vi "GOOP_ExecuteDependencyViewerCommand.vi"(10 "Object":u64, 11 "Sub Command":string) -> ()   [LabVIEW 2020]
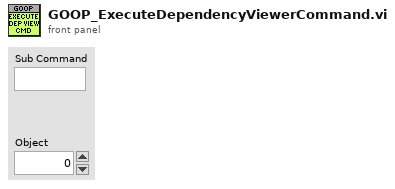
[diagram p1: front panel]
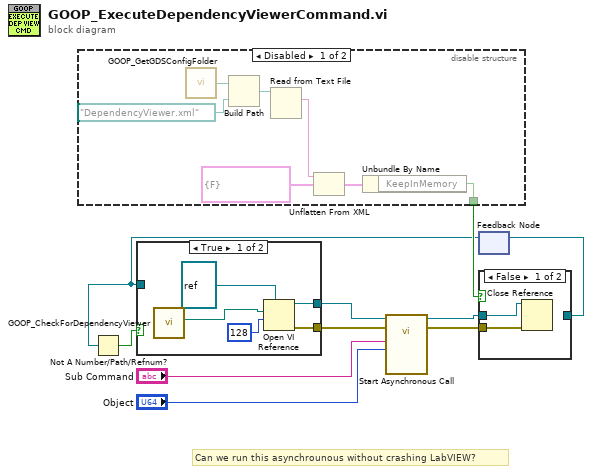
[diagram p0: block diagram]
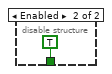
[diagram p2: hidden frame]
diagram:
  # "Can we run this asynchrounous without crashing LabVIEW?"
  n1 = disable-structure shown="Disabled" {
    disable-tunnel: [w11 TRUE ("KeepInMemory")] -> w4
    frame Disabled {
      n2 = call <resource>:"GOOP_GetGDSConfigFolder.vi"() -> ("GDSFolderPath"=w17:path)
      n3 = Build Path(base path=w17, name or relative path=path "DependencyViewer.xml") -> (appended path=w15:path)
      n4 = Read from Text File(file (use dialog)=w15) -> (text=w14:string)  [unwired: 3 in, 3 out]
      n5 = Unflatten From XML(xml string=w14, type=cluster{"KeepInMemory":bool} {"KeepInMemory"=FALSE}) -> (value=w12:cluster{"KeepInMemory":bool})  [unwired: 1 in, 1 out]
      n6 = Unbundle By Name(w12) -> ("KeepInMemory"=w11:bool)
    }
    frame Enabled {
    }
  }
  n7 = feedback #1() -> (w1:refnum<vi>)  [unwired: 1 in]
  n8 = Not A Number/Path/Refnum?(number/path/refnum=w1) -> (NaN/Path/Refnum?=w2:bool)
  n9 = case shown="True" w2 {
    tunnel: [w22 w24] -> w10
    tunnel: [w21 _] -> w9
    tunnel: w1 -> [_ w24]
    frame True {
      n10 = call <resource>:"GOOP_CheckForDependencyViewer.vi"() -> ("Dependency Viewer Path"=w19:path)  [unwired: 9 in, 2 out]
      n11 = Open VI Reference(type specifier VI Refnum (for type only)=refnum<vi> refnum, vi path=w19, options=128) -> (vi reference=w22:refnum<vi>, error out=w21:errorcluster)  [unwired: 3 in]
    }
    frame False {
    }
  }
  n12 = call-by-ref "Start Asynchronous Call"(reference=w10, error in=w9, "Object"="Object", "Sub Command"="Sub Command") -> (reference out=w6:refnum<vi>, error out=w5:errorcluster)  [unwired: 10 in]
  n13 = case shown="False" w4 {
    tunnel: w6 -> [w26 w27]
    tunnel: w5 -> [w25 _]
    tunnel: [_ w27] -> w3
    frame False {
      n14 = Close Reference(reference=w26, error in (no error)=w25) -> ()  [unwired: 1 out]
    }
    frame True {
    }
  }
  n15 = feedback-in #1(w3) -> ()
